vi "Set_IP_Simulation_Bit_Rate.vi"(8 "error in (no error)":errorcluster, 9 "Cellular Technology":T1="2G", 10 "value":i32=10 min=0 max=10, 11 "Base Station":T2) -> (0 "error out":errorcluster, 3 "Output String":string)   [LabVIEW 2021]
uses:
  Controls/Base_Station_Emulator.ctl
  Controls/Cellular_Technology.ctl
  Controls/TCP_FGV.ctl
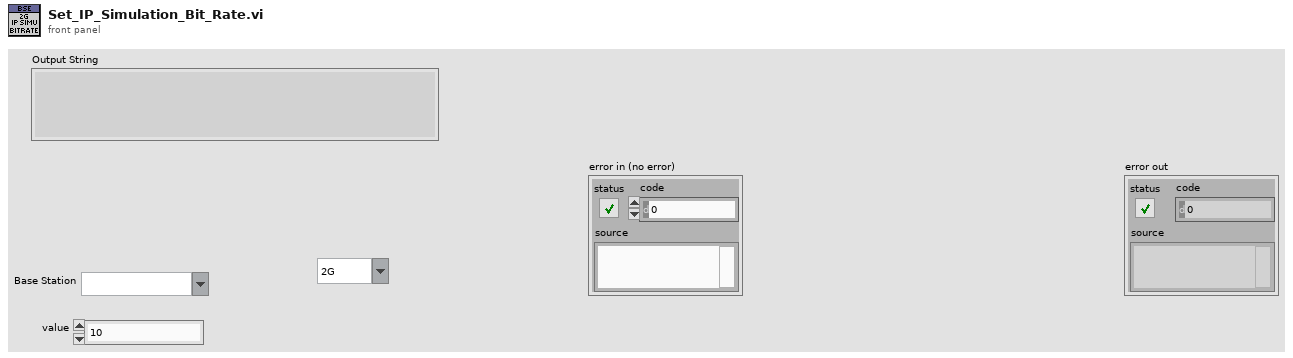
[diagram p1: front panel]
types:
  T1 = typedef "Cellular_Technology.ctl" = string
  T2 = typedef "Base_Station_Emulator.ctl" = string
  T3 = typedef "TCP_FGV.ctl" = enum16{"Open", "Read", "Write", "Close"}
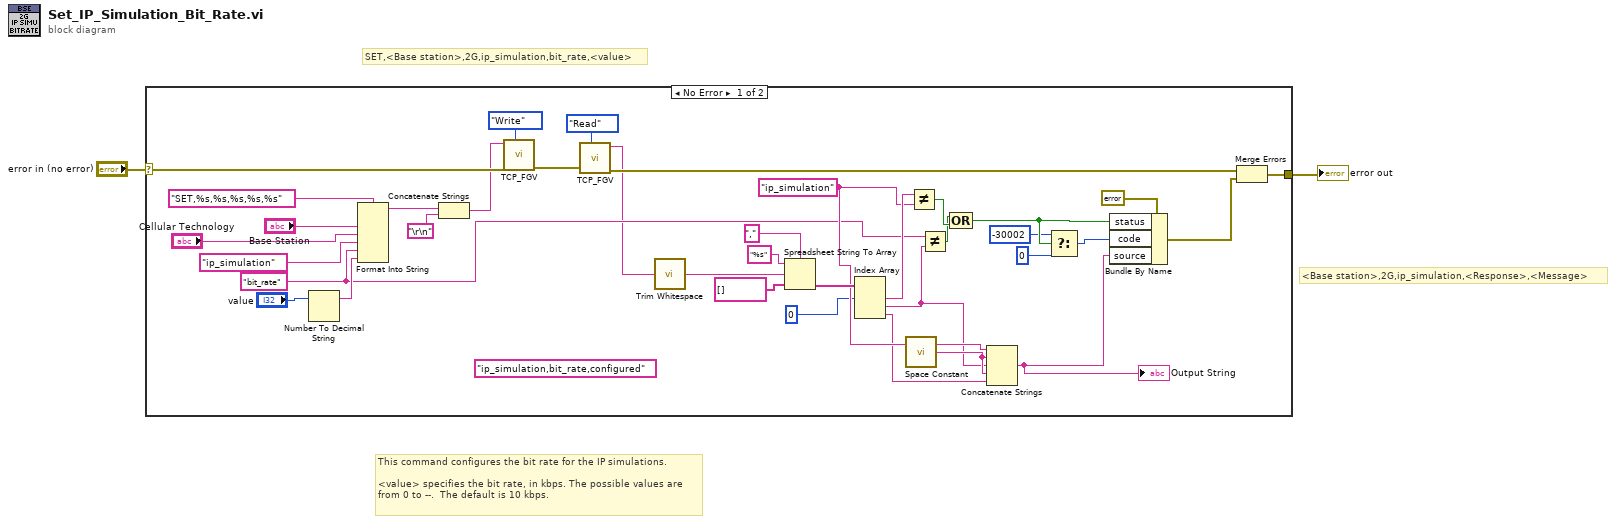
[diagram p0: block diagram]
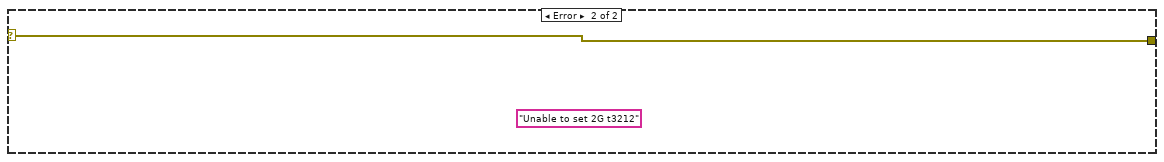
[diagram p2: hidden frame]
diagram:
  # "<Base station>,2G,ip_simulation,<Response>,<Message>"
  # "This command configures the bit rate for the IP simulations.\n \n<value> specifies the bit rate, in kbps. The possible values are\nfrom 0 to --.  The default is 10 kbps."
  # "SET,<Base station>,2G,ip_simulation,bit_rate,<value>"
  n1 = case shown="No Error" "error in (no error)" {
    selector: "error in (no error)" -> [w37 w40]
    tunnel: [w21 w40] -> w1
    frame No Error {
      (unwired) "ip_simulation,bit_rate,configured" ("format string")
      w11 = "ip_simulation" ("format string")
      w6 = "bit_rate"
      n2 = Number To Decimal String(number="value") -> (decimal integer string=w17:string)  [unwired: 1 in]
      n3 = Format Into String(format string="SET,%s,%s,%s,%s,%s", "Base Station", "Cellular Technology", "ip_simulation", w6, w17) -> (resulting string=w15:string)  [unwired: 2 in, 1 out]
      n4 = Concatenate Strings(w15, "\r\n") -> (w14:string)
      n5 = call "TCP_FGV.vi"("Command"=w14, "error in (no error)"=w37, "Operation"=TCP_FGV."Write") -> ("error out"=w22:errorcluster)  [unwired: 6 in, 1 out]
      n6 = call "TCP_FGV.vi"("error in (no error)"=w22, "Operation"=TCP_FGV."Read") -> ("Data Out"=w3:string, "error out"=w24:errorcluster)  [unwired: 7 in]
      n7 = call <vilib>:"Trim Whitespace.vi"("string"=w3) -> ("trimmed string"=w33:string)  [unwired: 1 in]
      n8 = Spreadsheet String To Array(delimiter (Tab)=",", format string="%s", spreadsheet string=w33, array type (2D Dbl)=string[] []) -> (array=w32:string[])
      n9 = Index Array(array=w32, index #1=0 ("index")) -> (element #1=w25:string, element #2=w7:string, element #3=w9:string)  [unwired: 2 in]
      n10 = call <vilib>:"Space Constant.vi"() -> ("String"=w10:string)
      n11 = Not Equal?(x=w25, y=w11) -> (x != y?=w8:bool)
      n12 = Not Equal?(x=w6, y=w7) -> (x != y?=w5:bool)
      n13 = Compound Arithmetic op=OR(w5, w8) -> (w34:bool)
      n14 = Concatenate Strings(w11, w10, w7, w10, w9) -> (w20:string)
      "Output String" <- w20
      n15 = Select(t=-30002 ("code"), s=w34, f=0 ("code")) -> (s? t:f=w35:i32)
      n16 = Bundle By Name(cluster=errorcluster {"status"=FALSE, "code"=0, "source"=""} ("error constant"), "status"=w34, "code"=w35, "source"=w20) -> (w23:errorcluster)
      n17 = Merge Errors(w24, w23) -> (w21:errorcluster)
    }
    frame Error {
      (unwired) "Unable to set 2G t3212" ("source")
    }
  }
  "error out" <- w1
